vi "servers.vi"(8 "error in (no error)":errorcluster, 11 "tcpServer in":refnum<class "TcpServer.lvclass">) -> (0 "error out":errorcluster, 3 "tcpServer out":refnum<class "TcpServer.lvclass">)   [LabVIEW 2018, in "TcpServer.lvclass"]
doc: "Init TCP Listener and then start TCP Server Loop. When TCP Server ends, close TCP Listener reference."
uses:
  TcpServer.lvclass
  TcpServer.lvclass/TcpServer.ctl
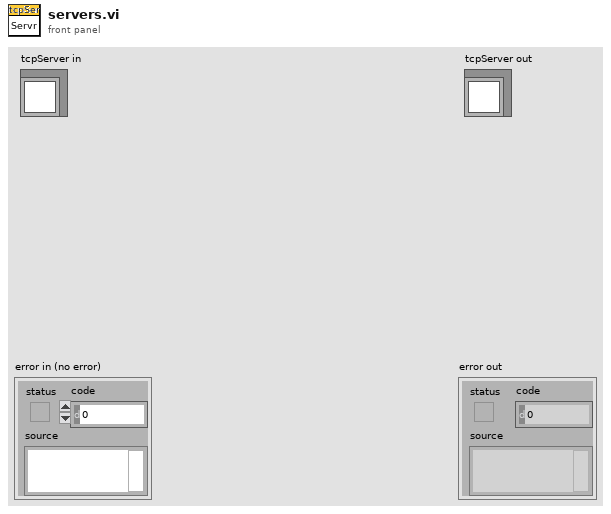
[diagram p1: front panel]
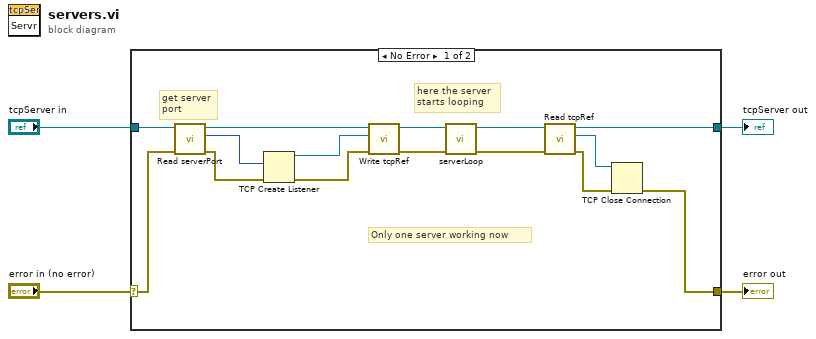
[diagram p0: block diagram]
diagram:
  n1 = case shown="No Error" "error in (no error)" {
    selector: "error in (no error)" -> [w17 w21]
    tunnel: [w5 w21] -> w3
    tunnel: [w10 w20] -> w1
    tunnel: "tcpServer in" -> [w19 w20]
    frame No Error {
      # "Only one server working now"
      # "here the server\nstarts looping"
      # "get server\nport"
      n2 = call "Read serverPort.vi"("error in (no error)"=w17, "tcpServer in"=w19) -> ("error out"=w8:errorcluster, "serverPort"=w18:u16, "tcpServer out"=w16:refnum<class "TcpServer.lvclass">)  [unwired: 7 in]
      n3 = TCP Create Listener(8:w8, 10:w18) -> (0:w7:errorcluster, 3:w14:refnum<k5>)  [unwired: 3 in, 1 out]
      n4 = call "Write tcpRef.vi"("error in (no error)"=w7, "tcpRef"=w14, "tcpServer in"=w16) -> ("error out"=w13:errorcluster, "tcpServer out"=w15:refnum<class "TcpServer.lvclass">)  [unwired: 7 in]
      n5 = call "serverLoop.vi"("error in (no error)"=w13, "tcpServer in"=w15) -> ("error out"=w11:errorcluster, "tcpServer out"=w12:refnum<class "TcpServer.lvclass">)  [unwired: 8 in]
      n6 = call "Read tcpRef.vi"("error in (no error)"=w11, "tcpServer in"=w12) -> ("error out"=w6:errorcluster, "tcpRef"=w9:refnum<k5>, "tcpServer out"=w10:refnum<class "TcpServer.lvclass">)  [unwired: 7 in]
      n7 = TCP Close Connection(connection ID=w9, error in (no error)=w6) -> (error out=w5:errorcluster)  [unwired: 1 in, 1 out]
    }
    frame Error {
    }
  }
  "error out" <- w3
  "tcpServer out" <- w1
